vi "Loop_ACT.vi"(10 "Camera Occurance":refnum<k4>) -> ()   [LabVIEW 2017, in "VisionHW.lvlib"]
uses:
  VisionHW.lvlib
  TypeDefs/CLUST_Targeting Data.ctl
  TypeDefs/CLUST_Cube Data.ctl
  TypeDefs/CLUST_Road Navigation Data.ctl
  TypeDefs/ENUM_Vision_Commands.ctl
  <vilib>/Rock Robotics/WPI/SerialPort/WPI_SerialPortRef.ctl
  _SHARE ALL/Global Share All/Global_STOP.vi
  Globals/Global_Vision_Data.vi
panel:
  out "Targeting Data":T1
  out "Target Data":string
  in  "Vision Command":string
  out "Cycle Time (S)":dbl format="%.3g"
  in  "Target Time(ms)":u32=50
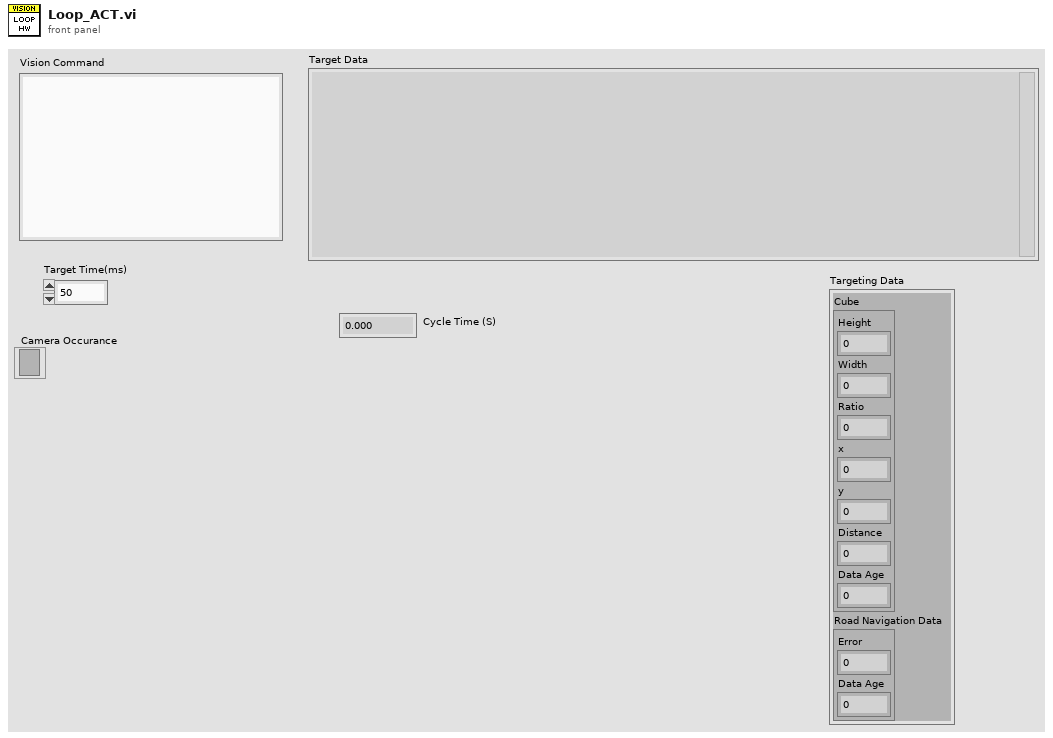
[diagram p1: front panel]
types:
  T1 = typedef "VisionHW.lvlib/CLUST_Targeting Data.ctl" = cluster{"Cube ":T2, "Road Navigation Data":T3}
  T2 = typedef "VisionHW.lvlib/CLUST_Cube Data.ctl" = cluster{"Height":dbl, "Width":dbl, "Ratio":dbl, "x":i32, "y":i32, "Distance ":i32, "Data Age":dbl}
  T3 = typedef "VisionHW.lvlib/CLUST_Road Navigation Data.ctl" = cluster{"Error":i32, "Data Age":dbl}
  T4 = typedef "WPI_SerialPortRef.ctl" = cluster{"DevStatus":errorcluster, "Serial Port Name":refnum<visa-resource-name>}
  T5 = typedef "ENUM_Vision_Commands.ctl" = enum16{"Init", "NoOp", "ResetCamera", "VideoOn", "VideoOff", "CubeDetection", "RoadNavigation"}
  T6 = cluster{"SerialRefOut":T4, " Log Output":string, "CMD":T5, "Target Time(ms)":u32, "Current Time":timestamp, "Previous Time":timestamp, "Cycle Time (S)":dbl, "Targeting Data":T1}
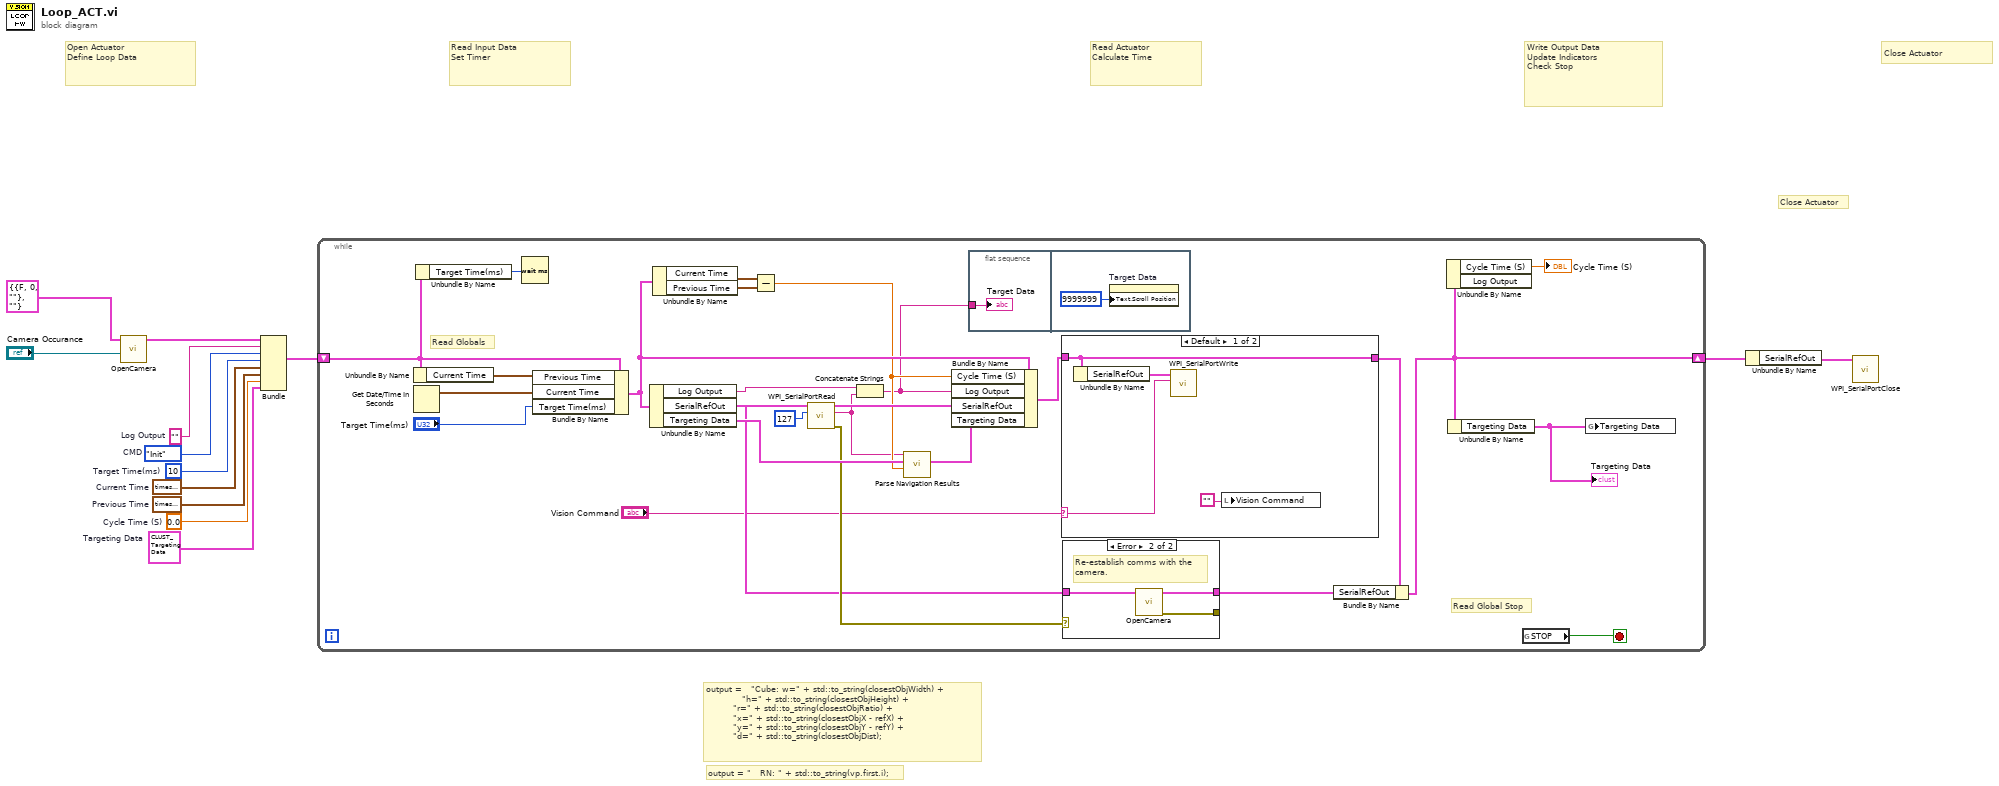
[diagram p0: block diagram]
diagram:
  w5 = T1 {"Cube "={"Height"=0.0, "Width"=0.0, "Ratio"=0.0, "x"=0, "y"=0, "Distance "=0, "Data Age"=0.0}, "Road Navigation Data"={"Error"=0, "Data Age"=0.0}}  # Targeting Data
  w8 = ENUM_Vision_Commands."Init"  # CMD
  w6 = 0.0  # Cycle Time (S)
  w13 = timestamp(0 s since 1904-01-01)  # Previous Time
  w12 = timestamp(0 s since 1904-01-01)  # Current Time
  w11 = u32 10  # Target Time(ms)
  w10 = ""  # Log Output
  # "output = \"   RN: \" + std::to_string(vp.first.i);"
  # "output =   \"Cube: w=\" + std::to_string(closestObjWidth) +\n\t\t   \t\t\t\t\t  \"h=\" + std::to_string(closestObjHeight) +\n\t\t\t\t\t\t\t  \"r=\" + std::to_string(closestObjRatio) +\n\t\t\t\t\t\t\t  \"x=\" + std::to_string(closestObjX - refX) +\n\t\t\t\t\t\t\t  \"y=\" + std::to_string(closestObjY - refY) +\n\t\t\t\t\t\t\t  \"d=\" + std::to_string(closestObjDist);"
  # "Close Actuator"
  # "Write Output Data\nUpdate Indicators\nCheck Stop"
  # "Read Actuator\nCalculate Time"
  # "Read Input Data\nSet Timer"
  # "Open Actuator\nDefine Loop Data"
  # "Close Actuator"
  n1 = call "OpenCamera.vi"("Camera Occurance"="Camera Occurance", "SerialPortRef"=T4 {"DevStatus"={"status"=FALSE, "code"=0, "source"=""}, "Serial Port Name"=""}) -> ("SerialRefOut"=w7:T4)  [unwired: 8 in, 1 out]
  n2 = Bundle("SerialRefOut"=w7, "Log Output"=w10, "CMD"=w8, "Target Time(ms)"=w11, "Current Time"=w12, "Previous Time"=w13, "Cycle Time (S)"=w6, "Targeting Data"=w5) -> (w4:T6)  [unwired: 1 in]
  n3 = while {
    shift-right: [w20] -> w9
    shift-left: w4 -> [w30]
    stop <- w39 stop-if-true
    # "Read Globals"
    # "Read Global Stop"
    n4 = Unbundle By Name(w30) -> ("Current Time"=w37:timestamp)
    n5 = Get Date/Time In Seconds() -> (seconds since 1Jan1904=w38:timestamp)
    n6 = Unbundle By Name(w30) -> ("Target Time(ms)"=w32:u32)
    n7 = Wait (ms)(milliseconds to wait=w32) -> ()  [unwired: 1 out]
    n8 = Bundle By Name(cluster=w30, "Previous Time"=w37, "Current Time"=w38, "Target Time(ms)"="Target Time(ms)") -> (w33:T6)
    n9 = Unbundle By Name(w33) -> ("Log Output"=w18:string, "SerialRefOut"=w28:T4, "Targeting Data"=w26:T1)
    n10 = Unbundle By Name(w33) -> ("Current Time"=w36:timestamp, "Previous Time"=w35:timestamp)
    n11 = Subtract(x=w36, y=w35) -> (x-y=w17:dbl)
    n12 = call <vilib>:"WPI_SerialPortRead.vi"("Num Bytes to Read"=u32 127 ("byte count"), "SerialPortRef"=w28) -> ("error out"=w23:errorcluster, "Buffer"=w14:string, "SerialPortRef"=w19:T4)  [unwired: 7 in]
    n13 = Concatenate Strings(w18, w14) -> (w15:string)
    n14 = call "Parse Navigation Results.vi"("Cycle Time"=w17, "Targeting Data In"=w26, "Target Data"=w14) -> ("Targeting Data Out"=w25:T1)  [unwired: 8 in]
    n15 = Bundle By Name(cluster=w33, "Cycle Time (S)"=w17, "Log Output"=w15, "SerialRefOut"=w19, "Targeting Data"=w25) -> (w27:T6)
    n16 = flat-sequence {
      tunnel: w15 -> [w44]
      frame #0 {
        "Target Data" <- w44
      }
      frame #1 {
        n17 = property on="Target Data" class="Str"("Text.Scroll Position"=u32 9999999) -> ()  [unwired: 2 in, 2 out]
      }
    }
    n18 = case shown="Default" "Vision Command" {
      selector: "Vision Command" -> [w46 _]
      tunnel: w27 -> [w49 w50]
      tunnel: [w49 w50] -> w22
      frame Default {
        n19 = Unbundle By Name(w49) -> ("SerialRefOut"=w48:T4)
        n20 = call <vilib>:"WPI_SerialPortWrite.vi"("Buffer"=w46, "SerialPortRef"=w48) -> ()  [unwired: 7 in, 3 out]
        n21 = local write "Vision Command"("") -> ()
      }
      frame "" {
      }
    }
    n22 = case shown="Error" w23 {
      tunnel: [_ w43] -> _
      tunnel: [w40 w42] -> w21
      tunnel: w19 -> [w40 w41]
      frame No Error {
      }
      frame Error {
        # "Re-establish comms with the\ncamera."
        n23 = call "OpenCamera.vi"("SerialPortRef"=w41) -> ("error out"=w43:errorcluster, "SerialRefOut"=w42:T4)  [unwired: 9 in]
      }
    }
    n24 = Bundle By Name(cluster=w22, "SerialRefOut"=w21) -> (w20:T6)
    n25 = Unbundle By Name(w20) -> ("Cycle Time (S)"=→"Cycle Time (S)":dbl)  [unwired: 1 out]
    n26 = Unbundle By Name(w20) -> ("Targeting Data"=w24:T1)
    "Targeting Data" <- w24
    n27 = global read "Global_STOP.vi" "STOP"() -> (w39:bool)
    n28 = global write "Global_Vision_Data.vi" "Targeting Data"(w24) -> ()
  }
  n29 = Unbundle By Name(w9) -> ("SerialRefOut"=w3:T4)
  n30 = call <vilib>:"WPI_SerialPortClose.vi"("SerialPortRef"=w3) -> ()  [unwired: 10 in, 1 out]
